vi "Dsitribute Central Message Handler Queue.vi"(8 "Error In":errorcluster, 11 "Dashboard In":refnum<class "Dashboard.lvclass">) -> (0 "Error Out":errorcluster, 3 "Dashboard Out":refnum<class "Dashboard.lvclass">)   [LabVIEW 2019, in "Dashboard.lvclass"]
uses:
  Dashboard.lvclass
  Accessors/Central Message Handler/Get Central Message Handler.vi
  Accessors/Processes/Get Processes.vi
  Central Message Handler/Accessors/Central Message Handler Queue/Get Central Message Handler Queue.vi
  Process/Accessors/Central Message Handler Queue/Set Central Message Handler Queue.vi
  Central Message Handler/Central Message Handler.lvclass
  Display Manager/Display Manager.lvclass
  Audio Analyzer/Audio Analyzer.lvclass
  Draw Frame/Draw Frame.lvclass
  Error Handling/Error Handling.lvclass
  Sequencer/Sequencer.lvclass
  Process/Process.lvclass
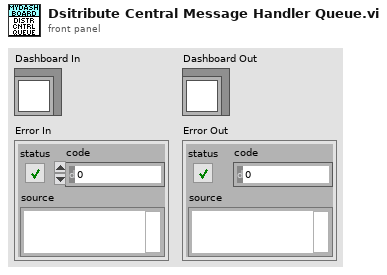
[diagram p1: front panel]
types:
  T1 = typedef "Dashboard.lvclass/Processes.ctl" = cluster{"Display Manager":refnum<class "Display Manager.lvclass">, "Audio Analyzer":refnum<class "Audio Analyzer.lvclass">, "Draw Frame":refnum<class "Draw Frame.lvclass">, "Error Handling":refnum<class "Error Handling.lvclass">, "Sequencer":refnum<class "Sequencer.lvclass">}
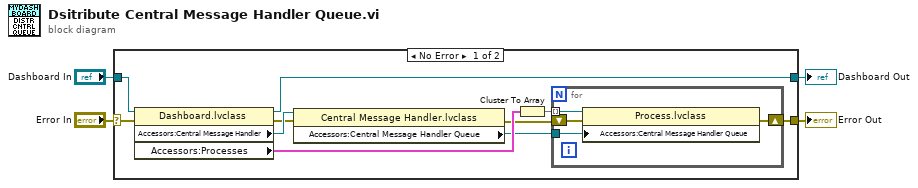
[diagram p0: block diagram]
diagram:
  n1 = case shown="No Error" "Error In" {
    selector: "Error In" -> [w13 w20]
    tunnel: [w14 w20] -> w4
    tunnel: [w11 w19] -> w3
    tunnel: "Dashboard In" -> [w12 w19]
    frame No Error {
      n2 = property class="Dashboard.lvclass"(reference=w12, error in=w13) -> (reference out=w11:refnum<class "Dashboard.lvclass">, error out=w7:errorcluster, "Accessors:Central Message Handler"=w8:refnum<class "Central Message Handler.lvclass">, "Accessors:Processes"=w9:T1)
      n3 = property class="Central Message Handler.lvclass"(reference=w8, error in=w7) -> (error out=w6:errorcluster, "Accessors:Central Message Handler Queue"=w5:refnum<queue>)  [unwired: 1 out]
      n4 = Cluster To Array(cluster=w9) -> (array=w10:refnum<class "Process.lvclass">[])
      n5 = for {
        tunnel: w10 -> [w16] mode=indexing
        shift-right: [w17] -> w14
        shift-left: w6 -> [w18]
        tunnel: w5 -> [w15]
        n6 = property class="Process.lvclass"(reference=w16, error in=w18, "Accessors:Central Message Handler Queue"=w15) -> (error out=w17:errorcluster)  [unwired: 1 out]
      }
    }
    frame Error {
    }
  }
  "Error Out" <- w4
  "Dashboard Out" <- w3
